vi "CliCreate.vi"(11 "error in (no error)":errorcluster) -> (4 "ref out":u64, 15 "error out":errorcluster)   [LabVIEW 2020, in "Snap7.lvlib"]
uses:
  Snap7.lvlib
  windows/lv_snap7.dll
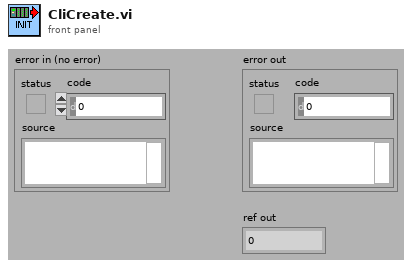
[diagram p1: front panel]
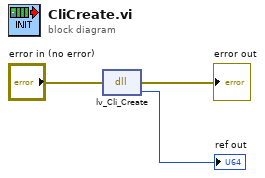
[diagram p0: block diagram]
diagram:
  n1 = dll-call lib="PTH2abs Dç¨åºä¸´æ¶ä¿®æ¹/180648-11æ»æå¼ålabview_è¿½æº¯ç2020-6-29SourcesOtherZLG_CANSnap7libwindowslv_snap7.dll" fn="lv_Cli_Create"(error in="error in (no error)") -> (error out=→"error out":errorcluster, "return type"=→"ref out":u64)  [unwired: 2 in, 1 out]
